vi "HRM-Stage4-close_main.vi"(8 "error in (no error)":errorcluster, 11 "Init cluster":T1) -> (0 "error out":errorcluster)   [LabVIEW 2020]
uses:
  HRM-Stage4-init_cluster.ctl
  HRM-Stage4-User_events.ctl
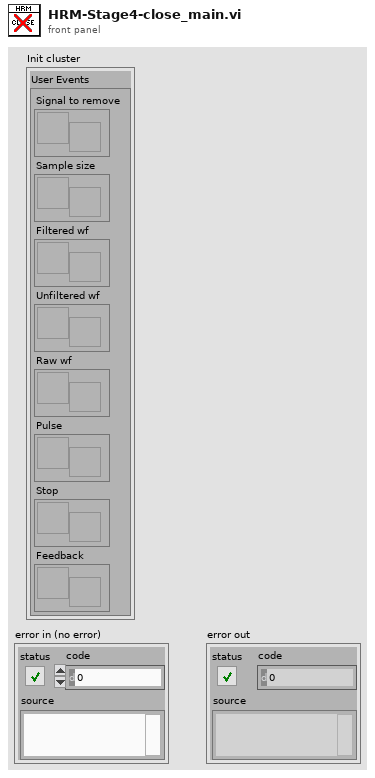
[diagram p1: front panel]
types:
  T1 = typedef "HRM-Stage4-init_cluster.ctl" = cluster{"User Events":T2}
  T2 = typedef "HRM-Stage4-User_events.ctl" = cluster{"Signal to remove":refnum<user-event>, "Sample size":refnum<user-event>, "Filtered wf":refnum<user-event>, "Unfiltered wf":refnum<user-event>, "Raw wf":refnum<user-event>, "Pulse":refnum<user-event>, "Stop":refnum<user-event>, "Feedback":refnum<user-event>}
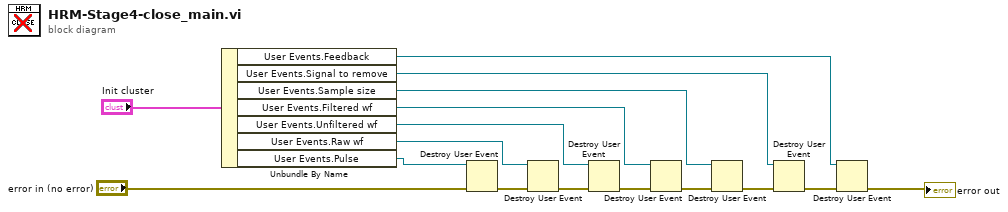
[diagram p0: block diagram]
diagram:
  n1 = Unbundle By Name("Init cluster") -> ("User Events.Feedback"=w2:refnum<user-event>, "User Events.Signal to remove"=w15:refnum<user-event>, "User Events.Sample size"=w14:refnum<user-event>, "User Events.Filtered wf"=w13:refnum<user-event>, "User Events.Unfiltered wf"=w12:refnum<user-event>, "User Events.Raw wf"=w11:refnum<user-event>, "User Events.Pulse"=w10:refnum<user-event>)
  n2 = Destroy User Event(user event=w10, error in="error in (no error)") -> (error out=w9:errorcluster)
  n3 = Destroy User Event(user event=w11, error in=w9) -> (error out=w5:errorcluster)
  n4 = Destroy User Event(user event=w12, error in=w5) -> (error out=w6:errorcluster)
  n5 = Destroy User Event(user event=w13, error in=w6) -> (error out=w7:errorcluster)
  n6 = Destroy User Event(user event=w14, error in=w7) -> (error out=w8:errorcluster)
  n7 = Destroy User Event(user event=w15, error in=w8) -> (error out=w4:errorcluster)
  n8 = Destroy User Event(user event=w2, error in=w4) -> (error out=→"error out":errorcluster)
